vi "Simple Controller test.vi"() -> ()   [LabVIEW 2017]
uses:
  <vilib>/Utility/inputDevices.llb/closeJoystick.vi
panel:
  out "error out":errorcluster
  out "sobot Driving Data Flat":string
  in  "stop":bool
  in  "error in (no error)":errorcluster
  in  "device index":i32
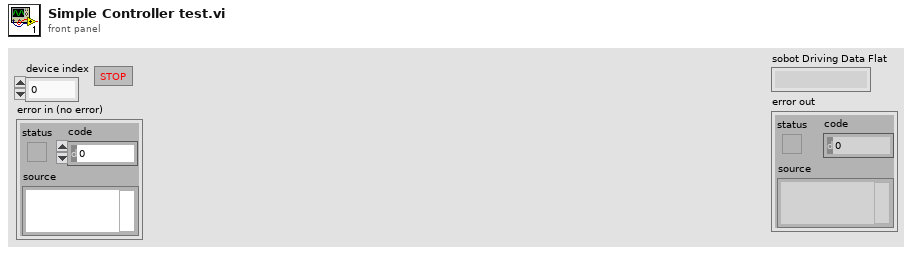
[diagram p1: front panel]
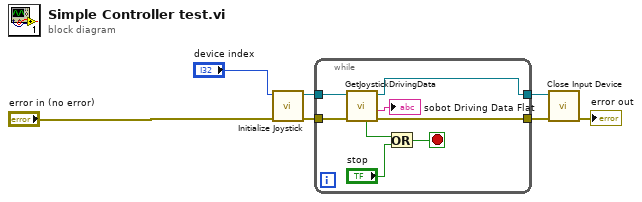
[diagram p0: block diagram]
diagram:
  n1 = call <vilib>:"Initialize Joystick.vi"("error in (no error)"="error in (no error)", "device index"="device index") -> ("error out"=w6:errorcluster, "device ID"=w7:refnum<k1>)  [unwired: 8 in]
  n2 = while {
    tunnel: w7 -> [w15]
    tunnel: w6 -> [w14]
    tunnel: [w12] -> w3
    tunnel: [w11] -> w2
    stop <- w8 stop-if-true
    n3 = call "GetJoystickDrivingData.vi"("error in (no error)"=w14, "Refnum in"=w15) -> ("error out"=w11:errorcluster, "data string"=→"sobot Driving Data Flat":string, "Refnum out"=w12:refnum<k1>, "Boolean"=w9:bool)  [unwired: 4 in, 2 out]
    n4 = Or(x=w9, y="stop") -> (x .or. y?=w8:bool)
  }
  n5 = call-poly <vilib>:"Close Input Device.vi"("error in (no error)"=w2, "device ID"=w3) -> ("error out"=→"error out":errorcluster)  [unwired: 8 in]
